vi "Get File Paths.vi"(8 "error in (no error)":errorcluster, 11 "Carya Config in":refnum<class "Carya Config.lvclass">) -> (0 "error out":errorcluster, 1 "Paths (all)":path[](array[path]), 2 "Path (1st)":path, 3 "Carya Config out":refnum<class "Carya Config.lvclass">)   [LabVIEW 2013, in "Carya Config.lvclass"]
doc: "Copyright 2018, Carya Automatisering, Wiebe Walstra."
uses:
  Carya Config.lvclass
  Carya Config.lvclass/Carya Config.ctl
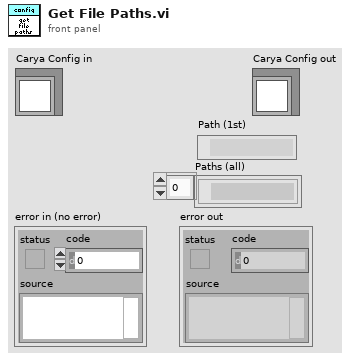
[diagram p1: front panel]
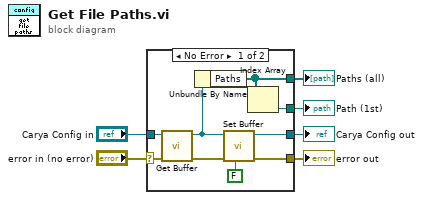
[diagram p0: block diagram]
diagram:
  n1 = case shown="No Error" "error in (no error)" {
    selector: "error in (no error)" -> [w15 w17]
    tunnel: [w10 w17] -> w5
    tunnel: [w9 w16] -> w3
    tunnel: "Carya Config in" -> [w14 w16]
    tunnel: [w13 _] -> w2
    tunnel: [w12 _] -> w1
    frame No Error {
      n2 = call-dynamic "Get Buffer.vi"("error in (no error)"=w15, "Carya Config in"=w14) -> ("error out"=w11:errorcluster, "Config"=w8:refnum<class "Carya Config.lvclass">)  [unwired: 8 in]
      n3 = Unbundle By Name(w8) -> ("Paths"=w12:path[])
      n4 = call-dynamic "Set Buffer.vi"("Set? [T]"=FALSE, "error in (no error)"=w11, "Carya Config"=w8) -> ("error out"=w10:errorcluster, "Carya Config out"=w9:refnum<class "Carya Config.lvclass">)  [unwired: 7 in]
      n5 = Index Array(array=w12) -> (element=w13:path)  [unwired: 1 in]
    }
    frame Error {
    }
  }
  "error out" <- w5
  "Carya Config out" <- w3
  "Path (1st)" <- w2
  "Paths (all)" <- w1
